vi "DestroyPublicEvents.vi"(8 "error in (no error)":errorcluster, 11 "Inst.Krohn-Hite-7008":refnum<class "Inst.Krohn-Hite-7008.lvclass">) -> (0 "error out":errorcluster, 3 "Inst.Krohn-Hite-7008 out":refnum<class "Inst.Krohn-Hite-7008.lvclass">)   [LabVIEW 2019, in "Inst.KH7008.lvlib" / "Inst.Krohn-Hite-7008.lvclass"]
doc: "JKI State Machine Objects (SMO) 1.0.0.5\nJKI - JKI\nCopyright (c) 2016, JKI"
uses:
  Inst.Krohn-Hite-7008.lvclass
  <userlib>/LevyLab/Instrument Framework/Instrument Types/Amplifier/Instrument.Amplifier.lvclass
panel:
  # "For instructions on how to use the JKI State Machine Objects, examples and video tutorials, visit:\nhttp://jki.net/state-machine-objects/\n\nJKI State Machine Objects™\nhttp://jki.net/state-machine-objects/\nCopyright (C) 2005-2015, JKI <info@jki.net>\nALL RIGHTS RESERVED"
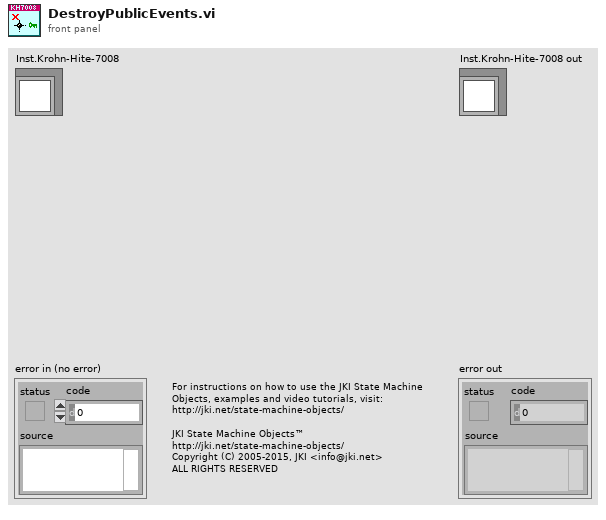
[diagram p1: front panel]
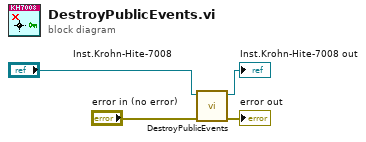
[diagram p0: block diagram]
diagram:
  n1 = call-parent "DestroyPublicEvents.vi"("error in (no error)"="error in (no error)", "Instrument"="Inst.Krohn-Hite-7008") -> ("error out"=→"error out":errorcluster, "Instrument out"=→"Inst.Krohn-Hite-7008 out":refnum<class "Inst.Krohn-Hite-7008.lvclass">)  [unwired: 8 in]
